vi "Test Opened Config Stays Closed on U32 Read.vi"(8 "error in (no error)":errorcluster, 11 "Test Case In":refnum<class "Configuration File Reference Management Test.lvclass">) -> (0 "error out":errorcluster, 3 "Test Case Out":refnum<class "Configuration File Reference Management Test.lvclass">)   [LabVIEW 2020, in "Configuration File Reference Management Test.lvclass"]
uses:
  Configuration File Reference Management Test.lvclass
  C:/Program Files (x86)/National Instruments/LabVIEW 2020/vi.lib/Astemes/LUnit/Test Case.lvclass
  Mock Configurable Base/Mock Configurable Base.lvclass
  <vilib>/Astemes/LUnit/Test Case.lvclass/Test Case.ctl
  <vilib>/Astemes/LUnit/Set Assertion Type.vi
  <vilib>/Astemes/LUnit/Palette/Pass.vi
  <vilib>/Astemes/LUnit/Palette/Fail.vi
  <vilib>/Astemes/LUnit/Add test result.vi
  <vilib>/Astemes/LUnit/LUnit Record Assertion Result.vi
  <vilib>/Astemes/LUnit/LUnit Aggregate Assertion Results.vi
  <vilib>/Astemes/LUnit/Method Result/LUnit Merge Status.vi
  <vilib>/Astemes/LUnit/LUnit Concatenate result strings.vi
  Configuration File Reference Management Test.lvclass/Configuration File Reference Management Test.ctl
  <vilib>/Astemes/LUnit/Test Case.lvclass
  C:/Git/astemes-triarc-framework/tests/Configuration File Reference Management Test/Configuration File Reference Management Test.lvclass
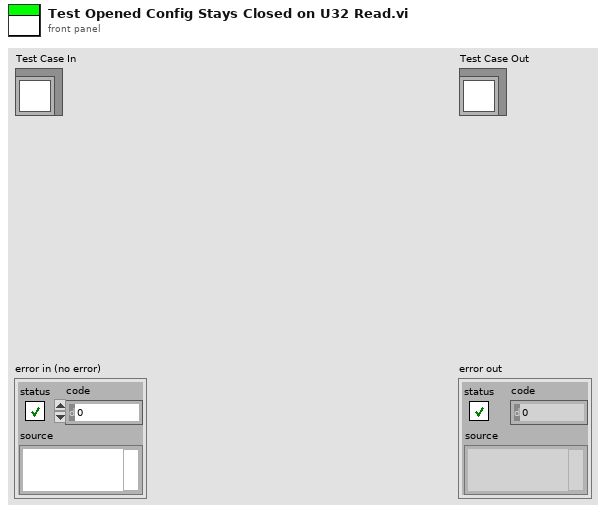
[diagram p1: front panel]
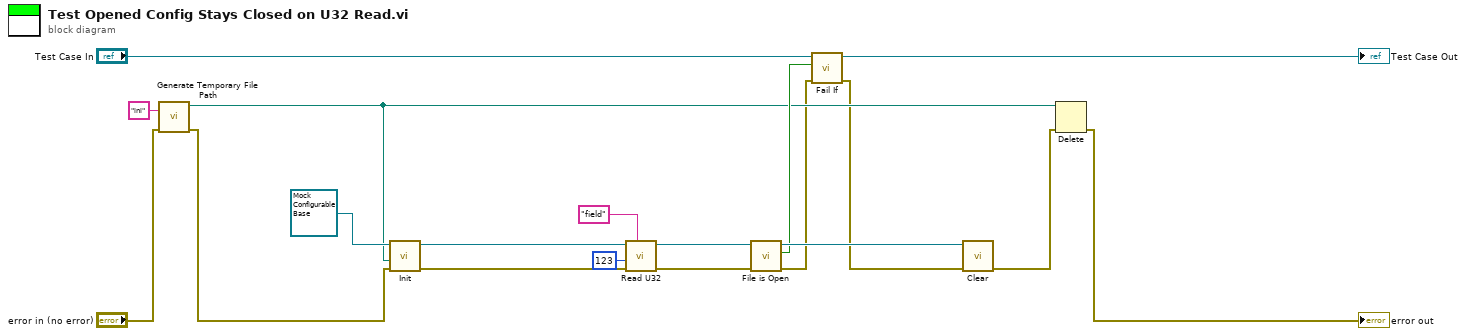
[diagram p0: block diagram]
diagram:
  n1 = call <vilib>:"Generate Temporary File Path.vi"("error in (no error)"="error in (no error)", "Temporary File Extension (tmp)"="ini") -> ("error out"=w17:errorcluster, "Unique Temporary File Path"=w6:path)  [unwired: 8 in]
  n2 = call-dynamic "Init.vi"("error in (no error)"=w17, "Config File Path"=w6, "Base In"=refnum<class "Mock Configurable Base.lvclass"> refnum ("Mock Configurable Base.lvclass")) -> ("error out"=w13:errorcluster, "Base Out"=w14:refnum<class "Mock Configurable Base.lvclass">)  [unwired: 7 in]
  n3 = call-dynamic "Read U32.vi"("key"="field", "error in (no error)"=w13, "default value"=u32 123 ("Value"), "Configuration File In"=w14) -> ("error out"=w12:errorcluster, "Configuration File Out"=w10:refnum<class "Mock Configurable Base.lvclass">)  [unwired: 5 in, 1 out]
  n4 = call "File is Open.vi"("error in (no error)"=w12, "Mock Configurable Base in"=w10) -> ("error out"=w3:errorcluster, "Is open?"=w7:bool, "Mock Configurable Base out"=w9:refnum<class "Mock Configurable Base.lvclass">)  [unwired: 7 in]
  n5 = call <vilib>:"Fail If.vi"("error in (no error)"=w3, "Fail?"=w7, "LUnit Test Case In"="Test Case In") -> ("error out"=w2:errorcluster, "LUnit Test Case Out"=→"Test Case Out":refnum<class "Configuration File Reference Management Test.lvclass">)  [unwired: 7 in]
  n6 = call-dynamic "Clear.vi"("error in (no error)"=w2, "Base In"=w9) -> ("error out"=w5:errorcluster)  [unwired: 9 in]
  n7 = Delete(path (use dialog)=w6, error in=w5) -> (error out=→"error out":errorcluster)  [unwired: 3 in, 2 out]
